vi "Module Loop.vi"(8 "error in (no error)":errorcluster, 11 "Sequence Submodule in":refnum<class "Sequence Submodule.lvclass">) -> (0 "error out":errorcluster, 3 "Sequence Submodule out":refnum<class "Sequence Submodule.lvclass">)   [LabVIEW 2020, in "VolatusSeq.lvlib" / "Sequence Submodule.lvclass"]
uses:
  Sequence Submodule.lvclass
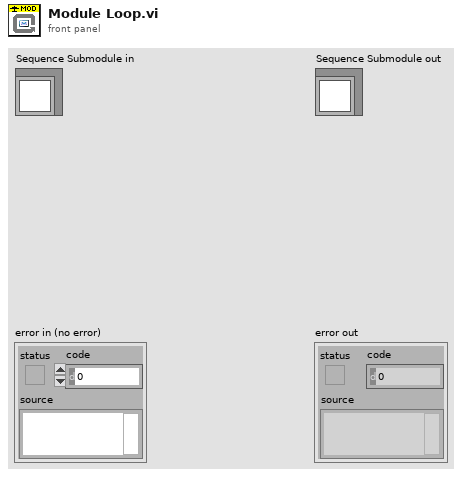
[diagram p1: front panel]
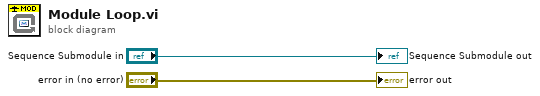
[diagram p0: block diagram]
diagram:
  "error out" <- "error in (no error)"
  "Sequence Submodule out" <- "Sequence Submodule in"
